vi "Global Setup.vi"(8 "error in (no error)":errorcluster, 11 "Demo Test in":refnum<class "Demo Test.lvclass">) -> (0 "error out":errorcluster)   [LabVIEW 2020, in "Demo Test.lvclass"]
uses:
  Demo Test.lvclass
  Demo Test.lvclass/Demo Test.ctl
  C:/git/astemes-lunit-global-fixture/source/Global Fixture Test Case/Global Fixture Test Case.lvclass
  C:/Program Files (x86)/National Instruments/LabVIEW 2020/vi.lib/Astemes/LUnit/Test Case.lvclass
  C:/Program Files (x86)/National Instruments/LabVIEW 2020/vi.lib/Astemes/LUnit/LUnit Runnable.lvclass
  C:/git/astemes-lunit-global-fixture/source/Demo Test/Demo Test.lvclass
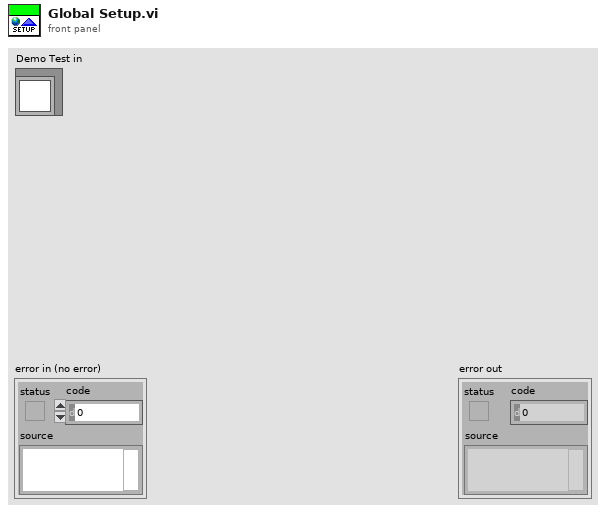
[diagram p1: front panel]
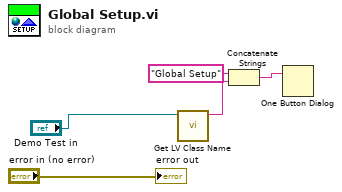
[diagram p0: block diagram]
diagram:
  n1 = call <vilib>:"Get LV Class Name.vi"("object"="Demo Test in") -> ("class name"=w1:string)  [unwired: 9 in, 1 out]
  n2 = Concatenate Strings("Global Setup" ("message"), w1) -> (w2:string)
  n3 = One Button Dialog(message=w2) -> ()  [unwired: 1 in, 1 out]
  "error out" <- "error in (no error)"
